vi "LocalizeFromImage.vi"(0 "tracker":u64, 1 "xcor_iterations":i32=2, 2 "input image":T1, 3 "debug image":T1) -> (6 "tracker":u64, 7 "COM":cluster{"comX":sgl, "comY":sgl}, 8 "debug image":T1(plugin-control), 9 "xcorpos":cluster{"XCor X":sgl, "XCor Y":sgl}, 10 "median":sgl)   [LabVIEW 2011]
uses:
  <vilib>/vision/Image Controls.llb/IMAQ Image.ctl
  TrackerDLL.vi
panel:
  in  "XCor X":sgl
  in  "XCor Y":sgl
  in  "comX":sgl
  in  "comY":sgl
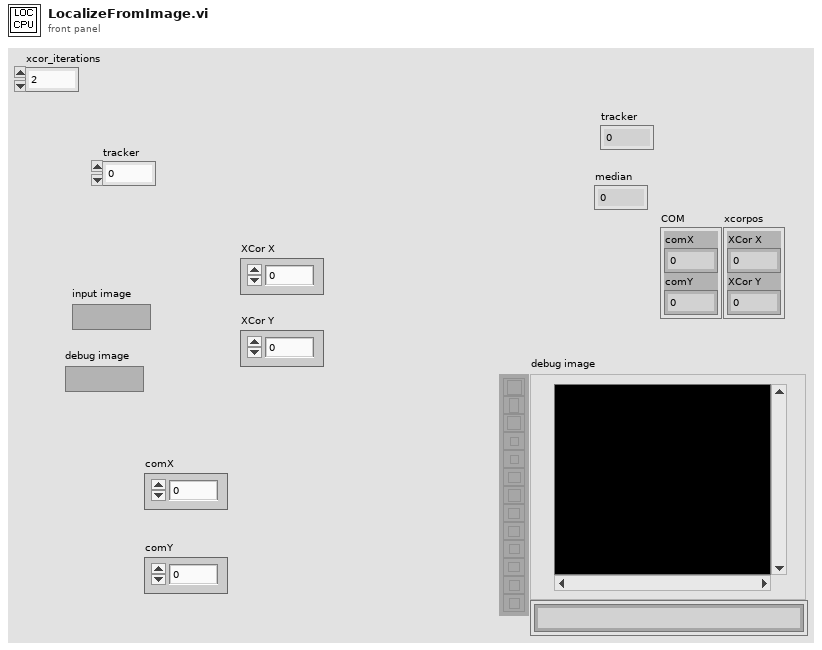
[diagram p1: front panel]
types:
  T1 = typedef "IMAQ Image.ctl" = refnum<image>
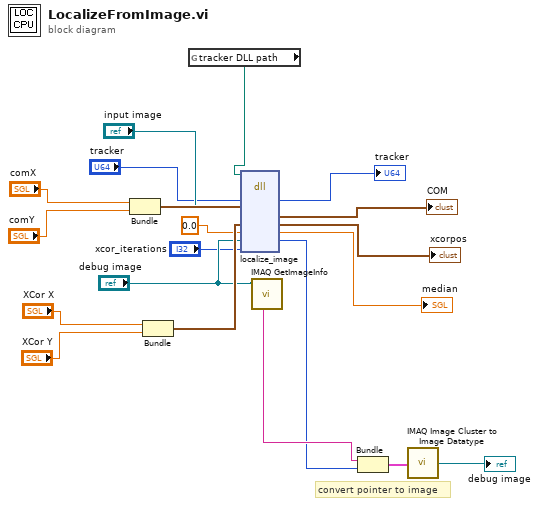
[diagram p0: block diagram]
diagram:
  # "convert pointer to image"
  n1 = Bundle("comX"="comX", "comY"="comY") -> (w18:cluster{"comX":sgl, "comY":sgl})  [unwired: 1 in]
  n2 = Bundle("XCor X"="XCor X", "XCor Y"="XCor Y") -> (w15:cluster{"XCor X":sgl, "XCor Y":sgl})  [unwired: 1 in]
  n3 = global read "TrackerDLL.vi" "tracker DLL path"() -> (w4:path)
  n4 = dll-call lib="D:/jcnossen1/cudaqi-tracker/Debug/cputrack.dll" fn="localize_image"(path in=w4, "tracker"="tracker", "image"="input image", "COM"=w18, "xcorpos"=w15, "median"=sgl 0.0, "debugImage"="debug image", "xcor_iterations"="xcor_iterations") -> ("tracker"=→"tracker":u64, "COM"=→"COM":cluster{"comX":sgl, "comY":sgl}, "xcorpos"=→"xcorpos":cluster{"XCor X":sgl, "XCor Y":sgl}, "median"=→"median":sgl, "debugImage"=w5:u64)  [unwired: 5 in, 2 out]
  n5 = call "IMAQ GetImageInfo"("Image"="debug image") -> ("Image Name"=w7:string)  [unwired: 3 in, 7 out]
  n6 = Bundle("Image Name"=w7, "debugImage"=w5) -> (w8:cluster{"Image Name":string, "debugImage":u64})  [unwired: 1 in]
  n7 = call <vilib>:"IMAQ Image Cluster to Image Datatype.vi"("Image"=w8) -> ("Image (dup)"=→"debug image":T1)
